vi "SamplesGenerated.vi"(3 "error in (no error)":errorcluster, 5 "task in":refnum<k24>) -> (0 "error out":errorcluster, 1 "SamplesGenerated":u32, 2 "task out":refnum<k24>)   [LabVIEW 2010]
uses:
  C:/Program Files/National Instruments/LabVIEW 2010/vi.lib/ULx/ULx_LV.dll
  Program Files/National Instruments/LabVIEW 2010/vi.lib/ULx/ULx_LV.dll
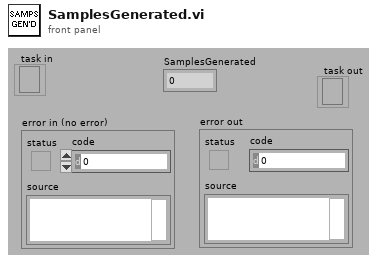
[diagram p1: front panel]
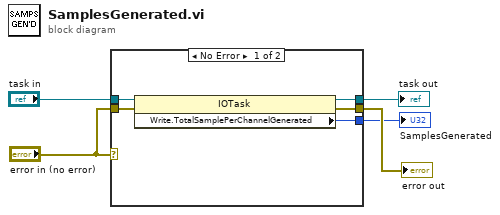
[diagram p0: block diagram]
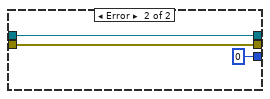
[diagram p2: hidden frame]
diagram:
  n1 = case shown="No Error" "error in (no error)" {
    tunnel: "task in" -> [w10 w13]
    tunnel: "error in (no error)" -> [w6 w12]
    tunnel: [w9 w13] -> w4
    tunnel: [w8 w12] -> w3
    tunnel: [w7 u32 0 ("Read.AvailableSamplePerChannel")] -> w1
    frame No Error {
      n2 = property class="IOTask"(reference=w10, error in=w6) -> (reference out=w9:refnum<k24>, error out=w8:errorcluster, "Write.TotalSamplePerChannelGenerated"=w7:u32)
    }
    frame Error {
    }
  }
  "task out" <- w4
  "error out" <- w3
  "SamplesGenerated" <- w1
